vi "Main.vi"(11 "Module Admin":refnum<class "Delacor_lib_QMH_Module Admin.lvclass">) -> ()   [LabVIEW 2021, in "Test Panel.lvlib"]
doc: "This template is based off of the Queued Message Handler design pattern and the Queued Message Handler project template that ships with LabVIEW.\n\nThe main difference is that the queue is private to this module and communication between modules is performed via Broadcast and Request events.\n\nRequest events are wrapped in public API methods and are handled in the Event Handling Loop (EHL) of this VI. Any module can register for Broadcast events sent by this module. The EHL generates messages based on user interface actions.\n\nThe Message Handling Loop (MHL) processes messages generated by the EHL, or by other messages. The messages are string values, so new messages can be added easily to the Message Cases case structure in the MHL. Each message cluster can also provide an optional value for Message Data, which is a variant that can be converted to whatever message-specific data is required.\n_____\nBased on DQMH Project Template 7.0.1.1316."
uses:
  Test Panel.lvlib
  <vilib>/Delacor/Delacor QMH/Libraries/Module Admin_class/Delacor_lib_QMH_Module Admin.lvclass
  Module Data--cluster.ctl
  GUI Ctrl Data's--Cluster.ctl
  Rx-Mapping Data.ctl
  <vilib>/Wovalab/Utilities/Helper Loop Periodic Timing/Helper Loop Periodic Timing.lvclass/Helper Loop Periodic Timing.ctl
  Host-Control's/Module ID Action Enum.ctl
  <vilib>/Delacor/Delacor QMH/Libraries/Message Queue_class/Delacor_lib_QMH_Message Queue.lvclass/Delacor_lib_QMH_Message Queue.ctl
  Digital Output/Controls/DO Update Cluster.ctl
  Stop Argument--cluster.ctl
  <vilib>/Delacor/Delacor QMH/Libraries/Module Admin_class/Delacor_lib_QMH_Module Admin.lvclass/Delacor_lib_QMH_Module Admin.ctl
  <vilib>/Utility/miscctls.llb/LVPointTypeDef.ctl
  Host-Control's/HW Name Enum.ctl
  <vilib>/Delacor/Delacor QMH/Libraries/Message Queue_class/Delacor_lib_QMH_Enqueue Message (Single).vi
  <vilib>/Delacor/Delacor QMH/Libraries/Module Admin_class/Delacor_lib_QMH_Get External Launch.vi
  <vilib>/Wovalab/Utilities/Helper Loop Periodic Timing/U32 Max Value--constant.vi
  <vilib>/Wovalab/Utilities/Helper Loop Periodic Timing/Update Last Execution Time.vi
  <vilib>/addons/_JKI.lib/Serialization/JSON/Library/Flatten To JSON String.vi
  <vilib>/Wovalab/Utilities/Helper Loop Periodic Timing/Helper Loop Periodic Timing.lvclass
  <vilib>/Delacor/Delacor QMH/Libraries/Message Queue_class/Delacor_lib_QMH_Message Queue.lvclass
  RT Acquisition Engine/RT Acquisition Engine.lvlib
  Main-Module/Host Main.lvlib
  <userlib>/_OpenG.lib/appcontrol/appcontrol.llb/openg_application_control.lvlib
  Hardware Selection/Hardware Selection.lvlib
  Test Panel GUI Update/Test Panel GUI Update.lvlib
panel:
  out "MFC Value's":T1
  out "Thermocouple Value's":T2
  out "AI-Channel Data's":dbl[](array[numeric])
  out "AI-Time":string
  out "AI-Channels":string[](array[string])
  out "Capsule-4":bool
  out "Capsule-3":bool
  out "Capsule-2":bool
  out "Time":string
  out "Data":bool[](array[boolean])
  out "Channels":string[](array[string])
  out "Drop Time":string
  in  "Gate valve Delay (mS)":u32=1000
  in  "EM valve Delay (mS)":u32=1000
  out "Auto Status":string
  out "12":dbl
  out "15":dbl
  out "16":dbl
  out "11":dbl
  out "14":dbl
  out "13":dbl
  out "8":dbl caption="Nichrome + S*2"
  out "7":dbl caption="Nichrome + S*1"
  out "6":dbl caption="Light S*2"
  out "10":dbl caption="Cam Trigger S*2"
  out "9":dbl caption="Cam Trigger S*1"
  out "5":dbl caption="Light S*1"
  out "4":dbl caption="Nichrome - S*2"
  out "3":dbl caption="Nichrome - S*1"
  out "2":dbl caption="Fan S*2"
  out "1":dbl caption="Fan S*1"
  in  "Sec Fan":bool
  out "Nicrome + 2":bool caption="Nichrome +"
  out "Current":dbl
  out "Diff":dbl
  out "Auto Seq":u8
  in  "Camera Trig. Delay(ms)":u32=50
  in  "Camera Trigger Delay(s)":bool=TRUE
  in  "Camera Power Off Delay(s)":u32
  out "Cam Trig from Release":bool
  out "Release Er No.":i32
  out "Safety Er No.":i32
  out "Proximity Status":string
  in  "Proximity_Disable":bool
  out "Status 2":string
  in  "Fan":bool
  in  "Cam Power":bool
  in  "Ground Clearance":dbl format="%#_13g"
  in  "Count down":dbl=7.0
  out "Pressure Signal 1":dbl format="%#_4g"
  out "Airbag Pressure":dbl format="%0#_4g"
  out "Gate Valve- Right 2":bool
  out "Gate Valve- Left":bool
  in  "Electro Magnet Lid-Right":bool
  in  "Electro Magnet Lid-Left":bool
  in  "Gate Valve-Left":bool
  in  "Gate Valve- Right":bool
  in  "Distance":dbl
  out "Ground Reference":dbl(slide) scale=0.0..500.0
  in  "Secondary Camera":bool
  in  "Motion Studio":bool
  in  "Stop":bool caption="Start_"
  out "NiCr Continuity":bool
  out "Safety":enum16{"Dis-Engaged by User", "Engaged"}(ring)
  out "Experimental":enum16{"Dis-Engaged by User", "Engaged"}(ring)
  out "Release":enum16{"Dis-Engaged by User", "Engaged"}(ring)
  out "SAFETY":bool
  out "RELEASE":bool
  out "SB-RIO":bool
  out "Capsule-1":bool
  out "Test Progress":bool
  out "Elapsed Time":dbl
  out "Message":string
  in  "Safety Valve_Switch":bool caption="Sensor power"
  in  "Check for Proceed":bool
  in  "Primary Camera":bool
  in  "Nicrome Status":bool
  in  "Saftey and Release":bool
  in  "Numeric":dbl
  out "Captured":bool
  out "Capture Time":timestamp
  out "Proximity 2":timestamp
  out "Start Time":timestamp
  out "Proximity":bool
  in  "Cam Trigger":bool
  in  "Nicrome -":bool caption="Nichrome -"
  in  "Nicrome +":bool caption="Nichrome +"
  in  "Light":bool
  in  "Sensor power":bool caption="Sensor Power"
  in  "Enable":bool
  out "Safety Sensor 3":bool
  out "Safety Sensor 2":bool
  out "Safety Sensor 1":bool
  out "Unlock Sensor":bool
  out "Lock Sensor":bool
  in  "Release Valve Control":bool caption="Sensor power"
  out "Valve 1":bool
  out "Valve 2":bool
  out "Valve 3":bool
  out "Release Valve":bool
  in  "Start":bool caption="Sensor power"
  out "Drag Shield Refernce":dbl(slide) scale=0.0..500.0
  out "error out 2":errorcluster
  out "error out":errorcluster
  out "Status":string
  in  "Simulate MHL Error":bool
  in  "Simulate EHL Error":bool
  # "IIT M Drop Tower Test System"
  # "MIMIC PANEL"
  # "STATUS"
  # "USER CHECK LIST"
  # "DROP CONTROL"
  # "Safety And Release"
  # "Circuit Status"
  # "Primary camera"
  # "Secondary camera"
  # "Check To Proceed"
  # "RELEASE"
  # "SAFETY"
  # "Experimental Capsule Parameters"
  # "DROP CAPSULE STATUS"
  # "AIRBAG CONTROLLER"
  # "Gate valve and Electromagnet Control"
  # "Gate valve Status"
  # "Pressure Indicator"
  # "In mm"
  # "m"
  # "In mm"
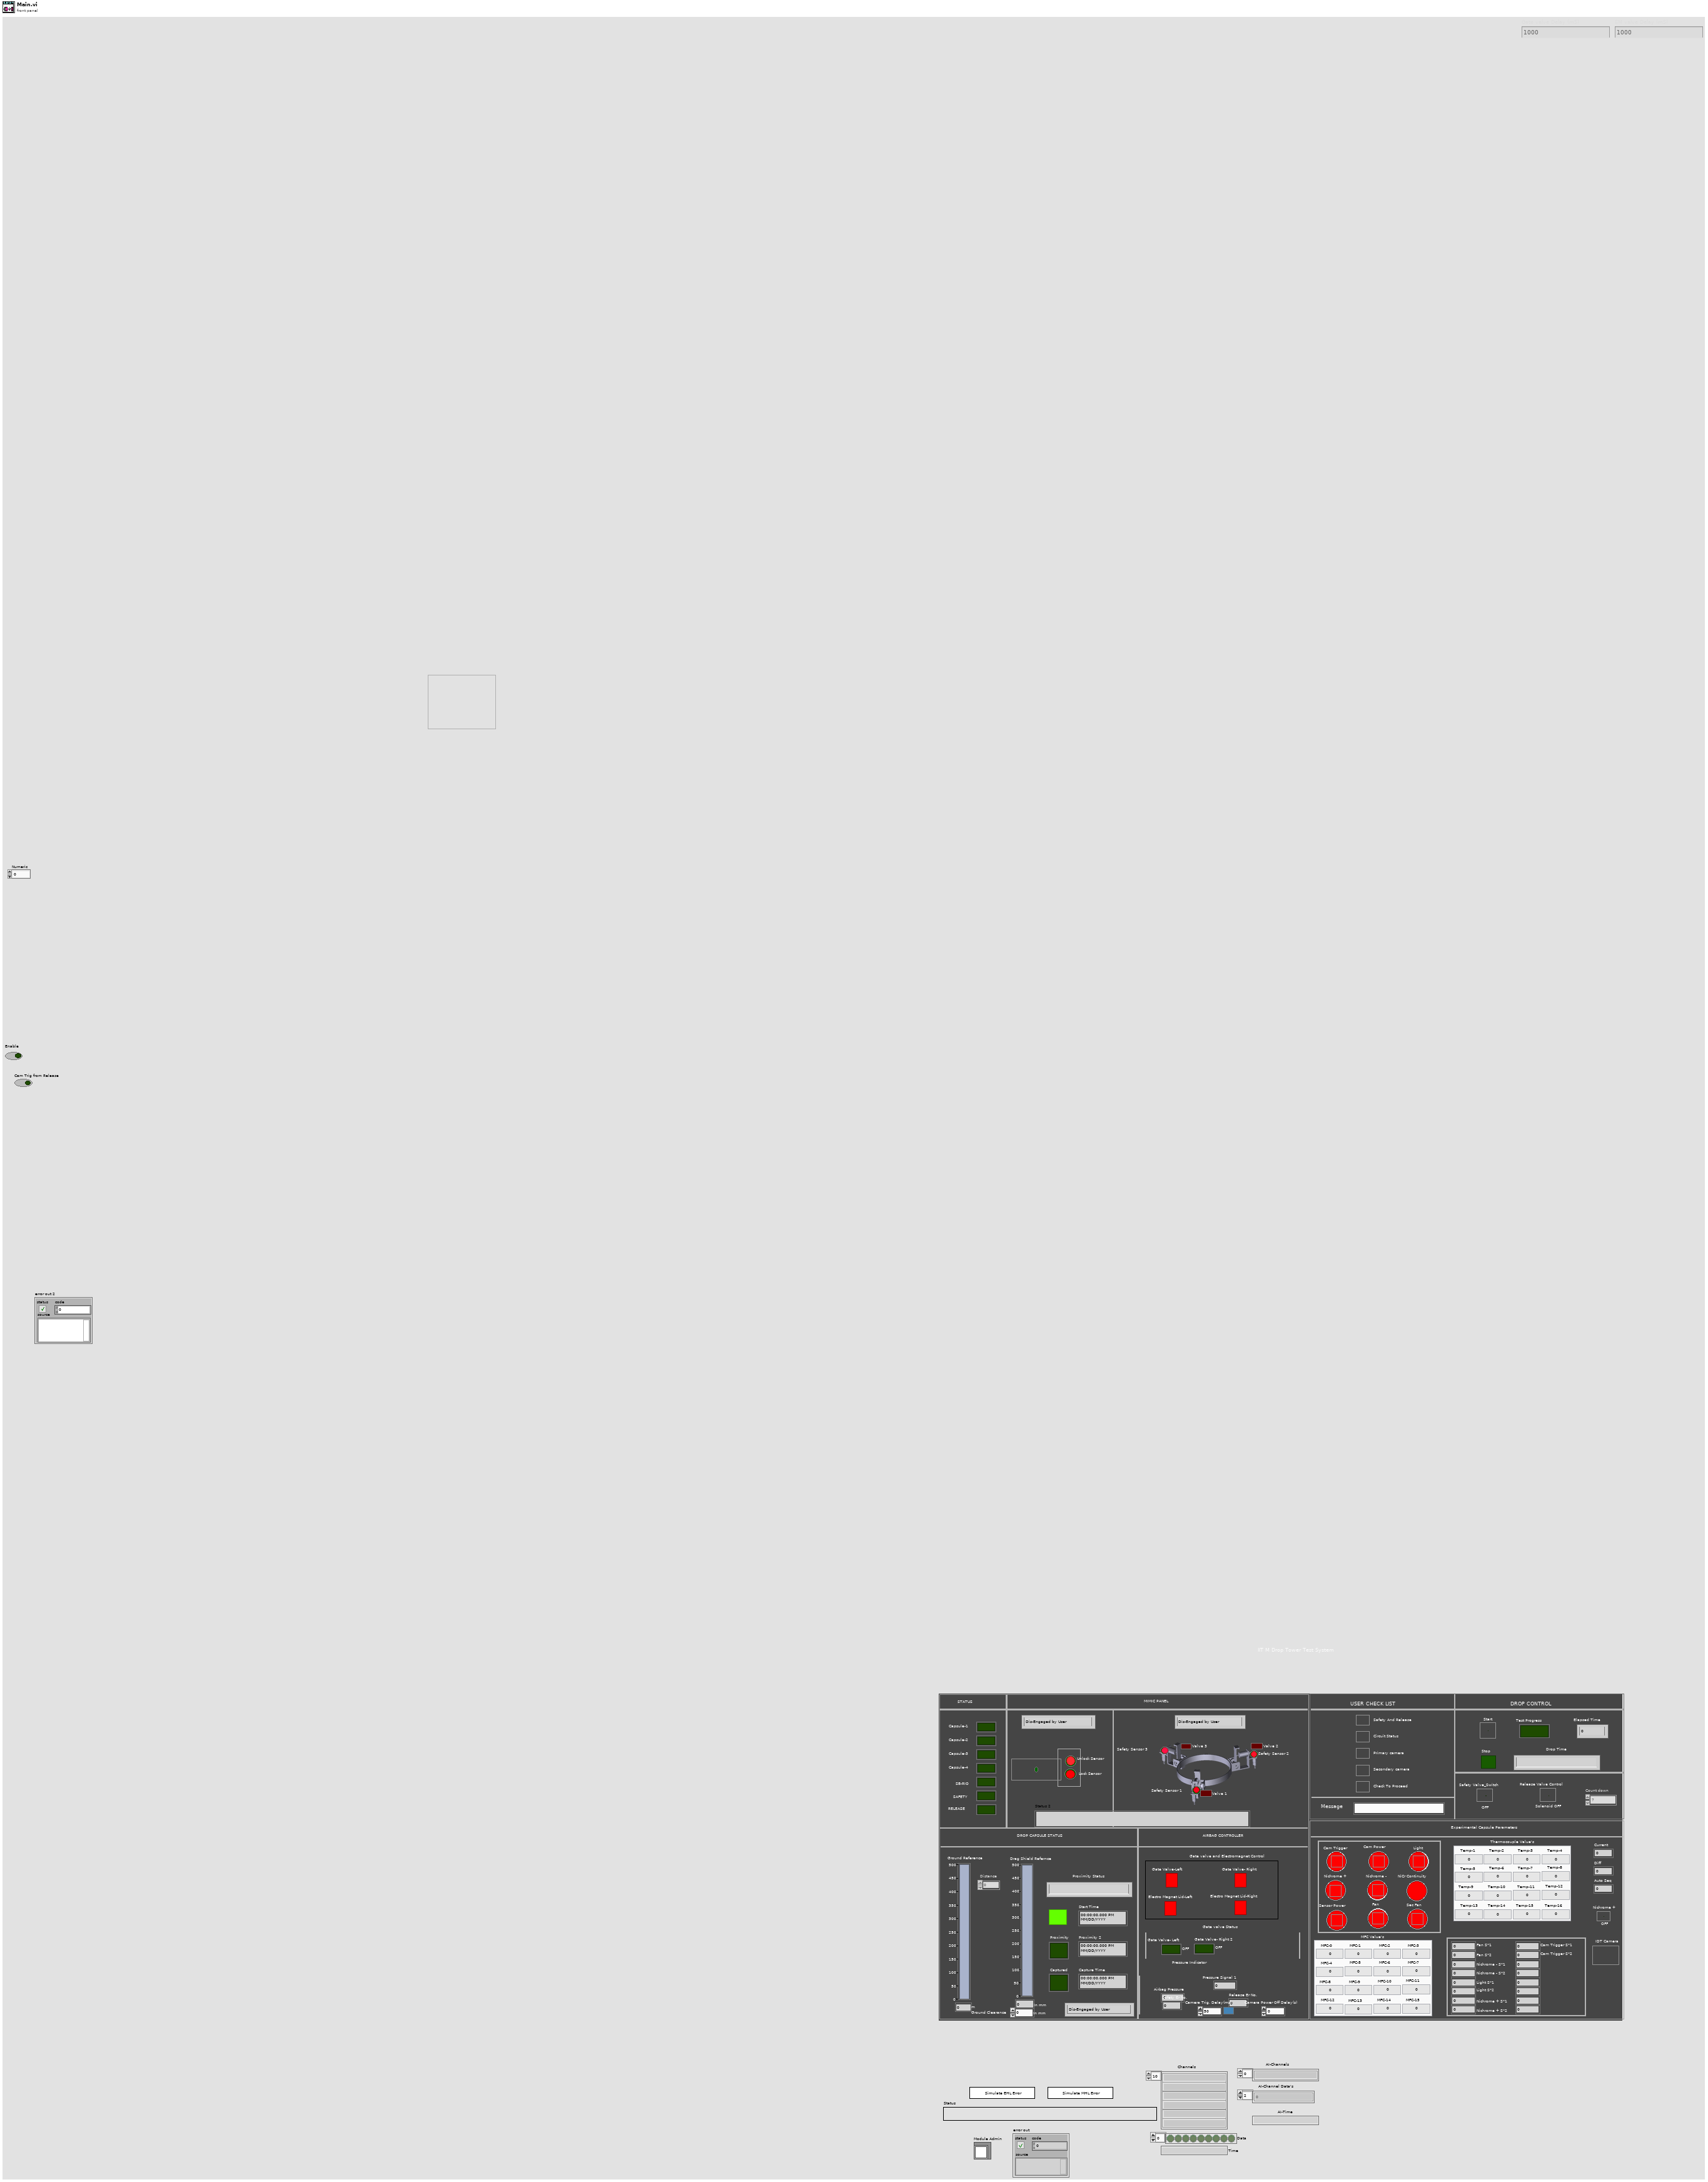
[diagram p1: front panel]
types:
  T1 = cluster{"MFC-0":dbl, "MFC-1":dbl, "MFC-2":dbl, "MFC-3":dbl, "MFC-4":dbl, "MFC-5":dbl, "MFC-6":dbl, "MFC-7":dbl, "MFC-8":dbl, "MFC-9":dbl, "MFC-10":dbl, "MFC-11":dbl, "MFC-12":dbl, "MFC-13":dbl, "MFC-14":dbl, "MFC-15":dbl}
  T2 = cluster{"Temp-1":dbl, "Temp-2":dbl, "Temp-3":dbl, "Temp-4":dbl, "Temp-5":dbl, "Temp-6":dbl, "Temp-7":dbl, "Temp-8":dbl, "Temp-9":dbl, "Temp-10":dbl, "Temp-11":dbl, "Temp-12":dbl, "Temp-13":dbl, "Temp-14":dbl, "Temp-15":dbl, "Temp-16":dbl}
  T3 = typedef "Test Panel.lvlib/Request Events--cluster.ctl" = cluster{"Stop Module":refnum<user-event>, "Show Panel":refnum<user-event>, "Hide Panel":refnum<user-event>, "Get Module Execution Status":refnum<user-event>, "Show Diagram":refnum<user-event>}
  T4 = typedef "Test Panel.lvlib/Module Data--cluster.ctl" = cluster{"Status":string, "RT-HW-Data":cluster{"RT-HW-Name":string[], "RT-HW-IP":string[]}, "Pane":refnum<vi>, "Tx-Maping Data":string[][], "GUI Ctrl Data's":T5, "Rx-Mapping Data":T6, "This VI":refnum<vi>}
  T5 = typedef "Test Panel.lvlib/GUI Ctrl Data's--Cluster.ctl" = cluster{"All Ctrl and Indi Label":string[], "All Ctrl & Indi Ref":refnum<vi>[]}
  T6 = typedef "Test Panel.lvlib/Rx-Mapping Data.ctl" = cluster{"Mapped Ctrl and Indi Label":string[], "Mapped Hardware Name":string[], "Mapped Interface Name":string[], "Mapped Channel Name":string[]}
  T7 = typedef "Module ID Action Enum.ctl" = enum16{"Init", "Insert", "Get a ID", "Get all ID"}
  T8 = cluster{"RT-HW-Name":string[], "RT-HW-IP":string[]}
  T9 = typedef "DO Update Cluster.ctl" = cluster{"Channel":string[], "Data":u8[]}
  T10 = enum32{"invalid lock state", "Not Locked", "Locked (No Password)", "Password-protected"}
  T11 = typedef "Test Panel.lvlib/Stop Argument--cluster.ctl" = cluster{"Origin":string, "Exit via Stop Module Req?":bool, "Wait for Module to stop?":bool}
  T12 = typedef "LVPointTypeDef.ctl" = cluster{"Horizontal":i16, "Vertical":i16}
  T13 = enum32{"Invalid", "Standard", "Closed", "Hidden", "Minimized", "Maximized"}
  T14 = typedef "HW Name Enum.ctl" = enum16{"Capsule-1", "Capsule-2", "Capsule-3", "Capsule-4", "sb-RIO", "Safety", "Release"}
  T15 = typedef "Test Panel GUI Update.lvlib/Broadcast Events--cluster.ctl" = cluster{"Module Did Init":refnum<user-event>, "Status Updated":refnum<user-event>, "Error Reported":refnum<user-event>, "Module Did Stop":refnum<user-event>, "Update Module Execution Status":refnum<user-event>}
  T16 = typedef "RT Acquisition Engine.lvlib/Broadcast Events--cluster.ctl" = cluster{"Module Did Init":refnum<user-event>, "Status Updated":refnum<user-event>, "Error Reported":refnum<user-event>, "Module Did Stop":refnum<user-event>, "Update Module Execution Status":refnum<user-event>, "RT Connection Status":refnum<user-event>, "Tx RT Hardware Info":refnum<user-event>, "DO Data's":refnum<user-event>, "AI-Info":refnum<user-event>}
  T17 = typedef "Host Main.lvlib/Broadcast Events--cluster.ctl" = cluster{"Module Did Init":refnum<user-event>, "Status Updated":refnum<user-event>, "Error Reported":refnum<user-event>, "Module Did Stop":refnum<user-event>, "Update Module Execution Status":refnum<user-event>, "RT-Module Id's":refnum<user-event>}
  T18 = typedef "Hardware Selection.lvlib/Broadcast Events--cluster.ctl" = cluster{"Module Did Init":refnum<user-event>, "Status Updated":refnum<user-event>, "Error Reported":refnum<user-event>, "Module Did Stop":refnum<user-event>, "Update Module Execution Status":refnum<user-event>, "Selected RT HW":refnum<user-event>}
  T19 = typedef "DIO Data's from RT.ctl" = cluster{"Channels":string[], "Data":bool[], "Time":string}
  T20 = typedef "AI-Data from RT.ctl" = cluster{"Channel Name's":string[], "Channel Data's":dbl[], "Date & Time":string}
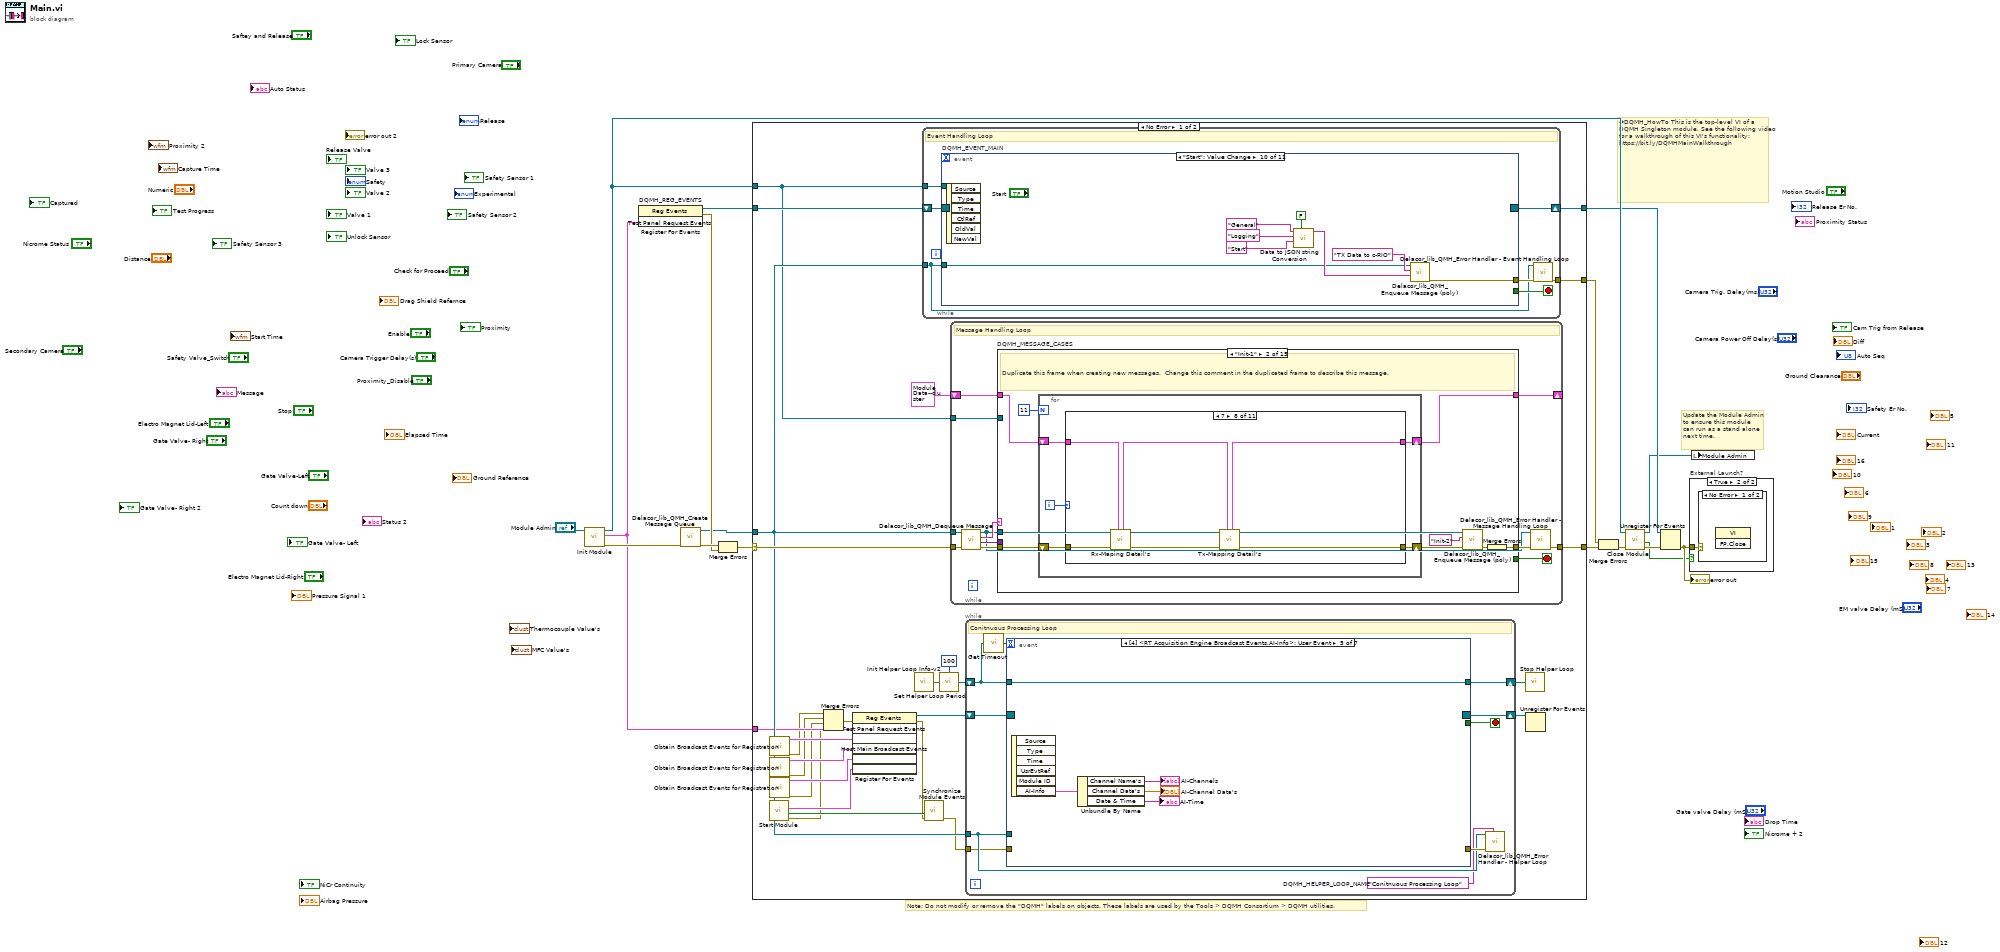
[diagram p0: block diagram]
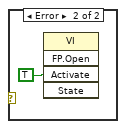
[diagram p3: hidden frame]
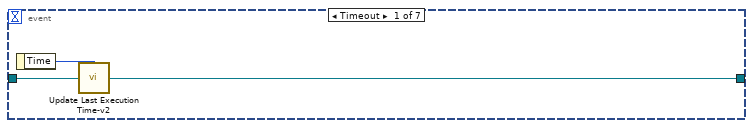
[diagram p4: hidden frame]
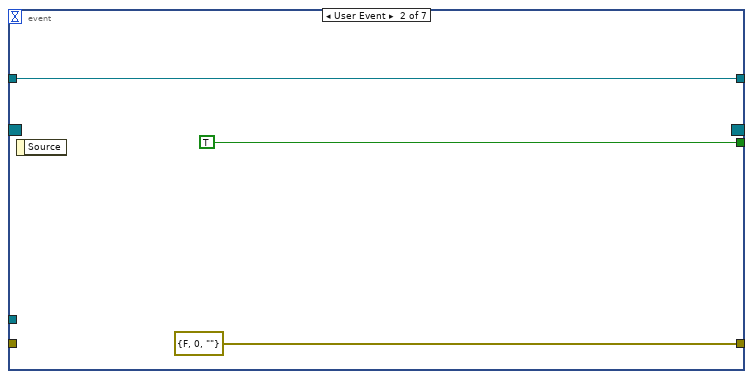
[diagram p5: hidden frame]
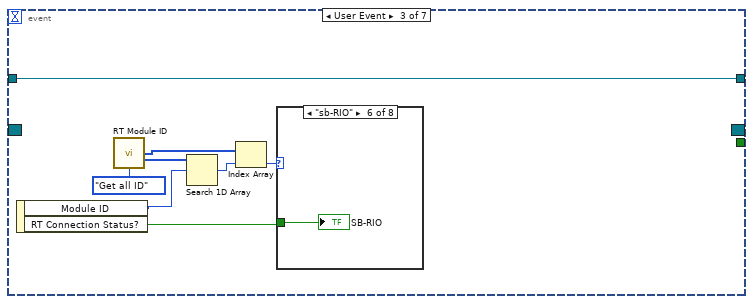
[diagram p6: hidden frame]
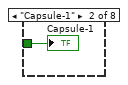
[diagram p8: hidden frame]
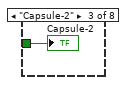
[diagram p9: hidden frame]
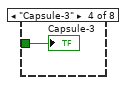
[diagram p10: hidden frame]
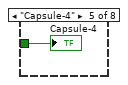
[diagram p11: hidden frame]
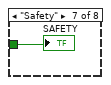
[diagram p12: hidden frame]
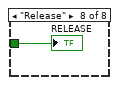
[diagram p13: hidden frame]
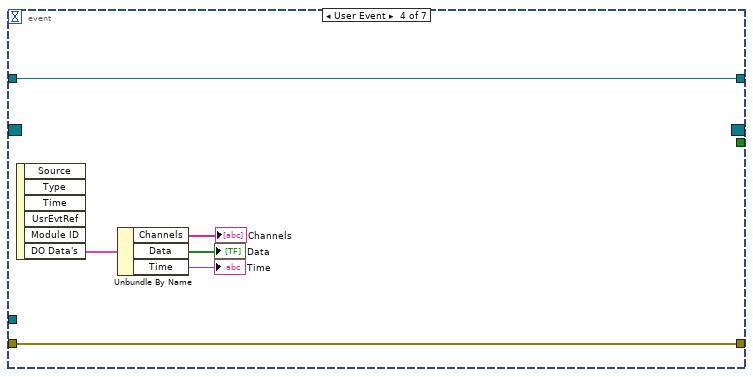
[diagram p14: hidden frame]
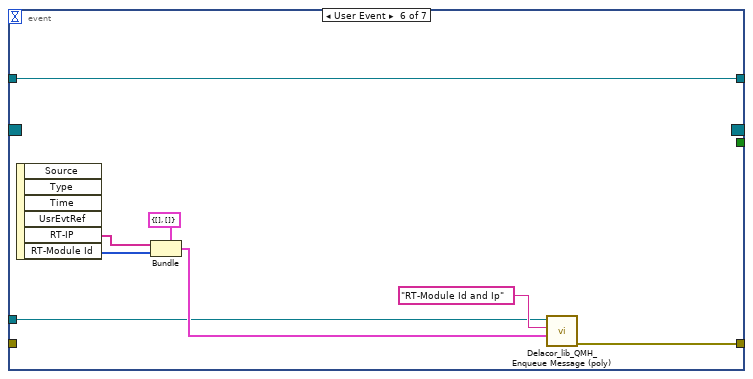
[diagram p15: hidden frame]
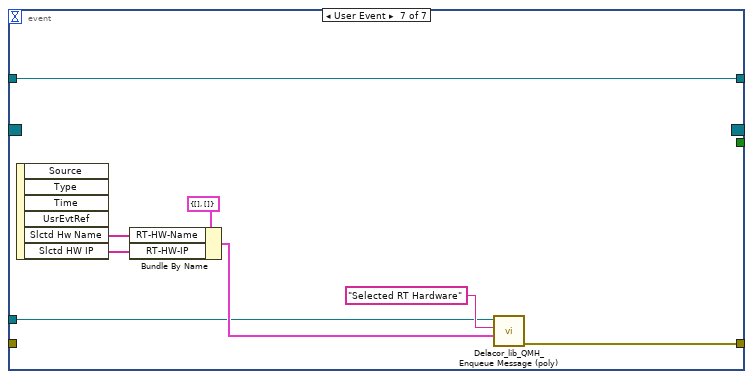
[diagram p16: hidden frame]
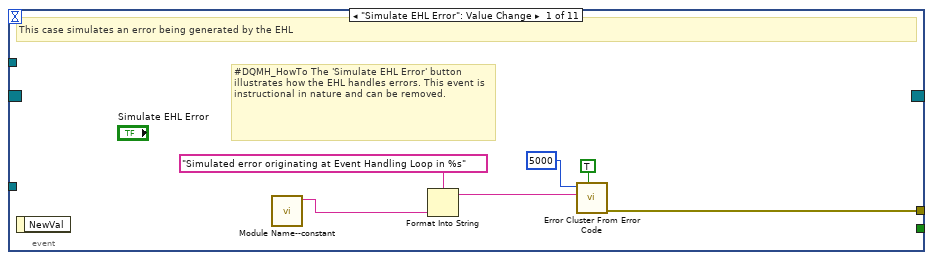
[diagram p17: hidden frame]
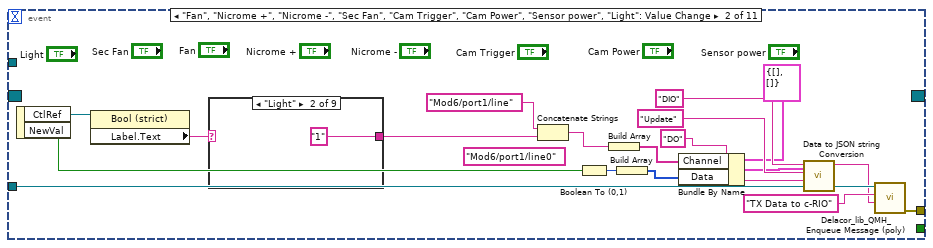
[diagram p18: hidden frame]
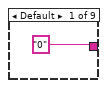
[diagram p19: hidden frame]
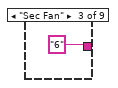
[diagram p20: hidden frame]
diagram:
  # "#DQMH_HowTo This is the top-level VI of a DQMH Singleton module. See the following video for a walkthrough of this VI's functionality: https://bit.ly/DQMHMainWalkthrough"
  # "Note: Do not modify or remove the \"DQMH\" labels on objects. These labels are used by the Tools > DQMH Consortium > DQMH utilities."
  # "Update the Module Admin to ensure this module can run as a stand alone next time."
  n1 = call "Init Module.vi"("Singleton Module Admin in"="Module Admin") -> ("error out"=w16:errorcluster, "Test Panel Request Events"=w1:T3, "Singleton Module Admin out"=w8:refnum<class "Delacor_lib_QMH_Module Admin.lvclass">)  [unwired: 8 in]
  n2 = register-events "DQMH_REG_EVENTS"(w1) -> (reference out=w6:refnum<event-registration>, error out=w9:errorcluster)  [unwired: 2 in]
  n3 = call <vilib>:"Delacor_lib_QMH_Create Message Queue.vi"("error in"=w16) -> ("error out"=w11:errorcluster, "Message Queue"=w5:refnum<class "Delacor_lib_QMH_Message Queue.lvclass">)  [unwired: 9 in]
  n4 = Merge Errors(w11, w9) -> (w10:errorcluster)
  n5 = case shown="No Error" w10 {
    selector: w10 -> [w42 w409]
    tunnel: [w44 w408] -> w17
    tunnel: [w41 w407] -> w7
    tunnel: w6 -> [w39 w407]
    tunnel: w5 -> [w38 w402]
    tunnel: [w43 _] -> w14
    tunnel: w8 -> [w37 w403]
    tunnel: w1 -> [w36 _]
    frame No Error {
      n6 = call "Start Module.vi"() -> ("error out"=w18:errorcluster, "Wait for Event Sync?"=w25:bool, "Test Panel GUI Update Broadcast Events"=w26:T15)  [unwired: 8 in, 1 out]
      n7 = call "Obtain Broadcast Events for Registration.vi"() -> ("error out"=w21:errorcluster, "RT Acquisition Engine Broadcast Events"=w29:T16)  [unwired: 9 in, 1 out]
      n8 = call "Obtain Broadcast Events for Registration.vi"() -> ("error out"=w20:errorcluster, "Host Main Broadcast Events"=w28:T17)  [unwired: 9 in, 1 out]
      n9 = call "Obtain Broadcast Events for Registration.vi"() -> ("error out"=w19:errorcluster, "Hardware Selection Broadcast Events"=w27:T18)  [unwired: 9 in, 1 out]
      n10 = Merge Errors(w21, w20, w19, w18) -> (w22:errorcluster)
      n11 = register-events ("DQMH_HELPER_REGFOREVENTS")(error in=w22, w36, w29, w28, w27, w26) -> (reference out=w34:refnum<event-registration>, error out=w24:errorcluster)  [unwired: 1 in]
      n12 = call <vilib>:"Init Helper Loop Info-v2.vi"() -> ("Helper Loop Periodic Timing"=w31:refnum<class "Helper Loop Periodic Timing.lvclass">)  [unwired: 1 in]
      n13 = while {
        tunnel: w38 -> [w103]
        shift-right: [w106] -> w41
        shift-left: w39 -> [w107]
        tunnel: [w108] -> w43
        tunnel: w37 -> [w104]
        stop <- w105 stop-if-true
        # "Event Handling Loop"
        n14 = event "DQMH_EVENT_MAIN" shown="[9] \"Start\": Value Change" {
          selector: w107 -> [_ _ _ _ _ _ _ _ _ _ _]
          dyn-events: [_ _ _ _ _ _ _ _ _ _ _] -> w106
          timeout: _ -> [_ _ _ _ _ _ _ _ _ _ _]
          tunnel: [_ _ _ _ _ _ _ TRUE ("Discard?") _ _ _] -> w105
          tunnel: w103 -> [_ w129 w144 _ _ _ _ w163 w180 w183 w193]
          tunnel: [w115 w130 w145 _ _ w151 _ w173 w181 w184 w195] -> w109
          tunnel: w104 -> [_ _ _ _ _ _ _ _ _ _ w192]
          event "Simulate EHL Error": Value Change {
            # "#DQMH_HowTo The 'Simulate EHL Error' button  illustrates how the EHL handles errors. This event is instructional in nature and can be removed."
            # "This case simulates an error being generated by the EHL"
            n15 = event-data() -> ()  [unwired: 1 in, 1 out]
            n16 = call "Module Name--constant.vi"() -> ("Module Name"=w112:string)  [unwired: 11 in]
            n17 = Format Into String(format string="Simulated error originating at Event Handling Loop in %s", w112) -> (resulting string=w113:string)  [unwired: 2 in, 1 out]
            n18 = call <vilib>:"Error Cluster From Error Code.vi"("show call chain? (False)"=TRUE, "error message (\"\")"=w113, "error code (0)"=5000) -> ("error out"=w115:errorcluster)  [unwired: 6 in]
          }
          event "Fan", "Nicrome +", "Nicrome -", "Sec Fan", "Cam Trigger", "Cam Power", "Sensor power", "Light": Value Change {
            (unwired) "Mod6/port1/line0" ("String")
            n19 = event-data() -> ("CtlRef"=w128:refnum<vi>, "NewVal"=w133:bool)  [unwired: 1 in]
            n20 = property class="Bool (strict)"(reference=w128) -> ("Label.Text"=w127:string)  [unwired: 1 in, 2 out]
            n21 = case shown="\"Light\"" w127 {
              tunnel: ["0" "1" "6" "5" "2" "3" "5" "4" "0"] -> w125
              frame Default {
              }
              frame "Light" {
              }
              frame "Sec Fan" {
              }
              frame "Fan" {
              }
              frame "Nicrome +" {
              }
              frame "Nicrome -" {
              }
              frame "Cam Trigger" {
              }
              frame "Cam Power" {
              }
              frame "Sensor power" {
              }
            }
            n22 = Concatenate Strings("Mod6/port1/line" ("String"), w125) -> (w124:string)
            n23 = Boolean To (0,1)(Boolean=w133) -> (0, 1=w132:i16)
            n24 = Build Array(w124) -> (w118:string[])
            n25 = Build Array(w132) -> (w117:i16[])
            n26 = Bundle By Name(cluster=T9 {"Channel"=[], "Data"=[]} ("DO Update Cluster"), "Channel"=w118, "Data"=w117) -> (w116:T9)
            n27 = call "Data to JSON string Conversion.vi"("Data"=w116, "SubCmd"="DO" ("Interface Data.SubCmd"), "Command"="Update" ("Interface Data.Command"), "Interface"="DIO") -> ("Cmd String"=w120:string)  [unwired: 6 in, 1 out]
            n28 = call-poly <vilib>:"Delacor_lib_QMH_Enqueue Message (poly).vi"("Message Data"=w120, "Message"="TX Data to c-RIO", "Message Queue in"=w129) -> ("error out"=w130:errorcluster)  [unwired: 7 in, 1 out]
          }
          event "Simulate MHL Error": Value Change {
            # "#DQMH_HowTo The 'Simulate MHL Error' button  illustrates how the MHL handles errors. This event is instructional in nature and can be removed."
            # "This case simulates an error being generated by the MHL"
            n29 = event-data() -> ()  [unwired: 1 in, 1 out]
            n30 = call-poly <vilib>:"Delacor_lib_QMH_Enqueue Message (poly).vi"("Message"="Simulate MHL Error", "Message Queue in"=w144) -> ("error out"=w145:errorcluster)  [unwired: 8 in, 1 out]
          }
          event User Event {
            # "Show the panel of this VI, and send a status updated message to let listeners know."
            # "Another Module called the \"Show Panel\" API Method."
            n31 = event-data() -> ()  [unwired: 1 in, 1 out]
            n32 = control-ref of="This VI"() -> (w147:refnum<vi>)
            n33 = call "Open VI Panel.vi"("VI"=w147) -> ()  [unwired: 10 in, 1 out]
            n34 = call "Status Updated.vi"("Status"="Panel shown." ("format string")) -> ()  [unwired: 10 in, 1 out]
          }
          event User Event {
            # "Hide the panel of this VI, and send a status updated message to let listeners know."
            # "Another Module called the \"Hide Panel\" API Method."
            n35 = event-data() -> ()  [unwired: 1 in, 1 out]
            n36 = control-ref of="This VI"() -> (w149:refnum<vi>)
            n37 = call "Hide VI Panel.vi"("VI"=w149) -> ()  [unwired: 10 in, 1 out]
            n38 = call "Status Updated.vi"("Status"="Panel hidden." ("format string")) -> ()  [unwired: 10 in, 1 out]
          }
          event User Event {
            # "Another Module called the \"Get Module Execution Status\" API Method."
            n39 = event-data() -> ()  [unwired: 1 in, 1 out]
            n40 = call "Update Module Execution Status.vi"("Running?"=TRUE) -> ("error out"=w151:errorcluster)  [unwired: 10 in]
          }
          event User Event {
            # "Another Module called the \"Show Diagram\" API Method. This event is used for debugging."
            n41 = event-data() -> ()  [unwired: 1 in, 1 out]
            n42 = disable-structure shown="RUN_TIME_ENGINE==False" {
              frame condition #0 (active) {
                # "functionality not available in exe"
                n43 = invoke on="Invoke Node" class="VI" method="Lock State.Get"() -> (error out=w157:errorcluster, "Get Lock State"=w156:T10, "pwd in cache"=w153:bool)  [unwired: 4 in, 1 out]
                n44 = Equal?(x=T10."Password-protected", y=w156) -> (x = y?=w154:bool)
                n45 = Compound Arithmetic op=AND(w154, invert w153) -> (w152:bool)
                n46 = case shown="False" w152 {
                  tunnel: w157 -> [w160 _]
                  frame False {
                    n47 = property on="Property Node" class="VI"(error in=w160, "BDWin.Open"=TRUE ("Block Diagram Window:Open")) -> ()  [unwired: 1 in, 2 out]
                    n48 = call "Status Updated.vi"("Status"="Block Diagram shown." ("format string")) -> ()  [unwired: 10 in, 1 out]
                  }
                  frame True {
                    # "Password-protected VI, and the password is not in the cache. Do not show the diagram."
                  }
                }
              }
              frame condition #1 {
              }
            }
          }
          event User Event {
            # "The Stop Module Event can get fired from the Exit message in the MHL. The queue gets destroyed in that case. If the queue no longer exists, the Enqueue Exit as a priority message will return error 1. It is safe to ignore, because the module is already exiting."
            # "Another Module called the \"Stop Module\" API Method  or the Message Handling Loop below."
            n49 = event-data() -> ("Origin"=w170:string, "Exit via Stop Module Req?"=w166:bool, "Wait for Module to stop?"=w165:bool)  [unwired: 1 in]
            n50 = local write "Status"(w170) -> ()
            n51 = Bundle By Name(cluster=T11 {"Origin"="", "Exit via Stop Module Req?"=FALSE, "Wait for Module to stop?"=FALSE} ("Stop Argument"), "Exit via Stop Module Req?"=w166, "Wait for Module to stop?"=w165) -> (w164:T11)
            n52 = call-dynamic "Delacor_lib_QMH_Flush Messages.vi"("Message Queue in"=w163) -> ("error out"=w161:errorcluster, "Message Queue out"=w162:refnum<class "Delacor_lib_QMH_Message Queue.lvclass">)  [unwired: 7 in, 2 out]
            n53 = call-poly <vilib>:"Delacor_lib_QMH_Enqueue Message (poly).vi"("Priority Message? (F)"=TRUE, "error in"=w161, "Message Data"=w164, "Message"="Exit", "Message Queue in"=w162) -> ("error out"=w174:errorcluster)  [unwired: 5 in, 1 out]
            n54 = call <vilib>:"Clear Errors.vi"("error in (no error)"=w174, "specific error code to clear (0: all)"=1) -> ("error out"=w173:errorcluster)  [unwired: 4 in, 1 out]
          }
          event "Release Valve Control": Value Change {
            n55 = event-data() -> ()  [unwired: 1 in, 3 out]
            n56 = call "Data to JSON string Conversion.vi"("Data"=FALSE, "SubCmd"="Start", "Command"="AutoSequence", "Interface"="General") -> ("Cmd String"=w179:string)  [unwired: 6 in, 1 out]
            n57 = call-poly <vilib>:"Delacor_lib_QMH_Enqueue Message (poly).vi"("Message Data"=w179, "Message"="TX Data to c-RIO", "Message Queue in"=w180) -> ("error out"=w181:errorcluster)  [unwired: 7 in, 1 out]
          }
          event "Start": Value Change {
            n58 = event-data() -> ()  [unwired: 1 in, 6 out]
            n59 = call "Data to JSON string Conversion.vi"("Data"=FALSE, "SubCmd"="Start", "Command"="Logging", "Interface"="General") -> ("Cmd String"=w189:string)  [unwired: 6 in, 1 out]
            n60 = call-poly <vilib>:"Delacor_lib_QMH_Enqueue Message (poly).vi"("Message Data"=w189, "Message"="TX Data to c-RIO", "Message Queue in"=w183) -> ("error out"=w184:errorcluster)  [unwired: 7 in, 1 out]
          }
          event Panel Close? {
            w194 = TRUE  # Discard the event, the MHL is responsible for closing and stopping this VI.
            # "Hide the panel or send the 'Exit' message if the user clicks the 'X' on the module main VI panel."
            n61 = event-data() -> ()  [unwired: 1 in, 1 out]
            n62 = property on="Property Node" class="Module Admin"(reference=w192) -> ("Accessors:External Launch"=w191:bool)  [unwired: 1 in, 2 out]
            n63 = case shown="False" w191 {
              tunnel: w193 -> [w201 w208]
              tunnel: [w197 w211] -> w195
              frame True {
                # "If externally launched, clicking the 'X' hides the panel, but doesn't close it."
                n64 = control-ref of="This VI"() -> (w205:refnum<vi>)
                n65 = call "Hide VI Panel.vi"("VI"=w205) -> ("error out"=w203:errorcluster)  [unwired: 10 in]
                n66 = call "Status Updated.vi"("error in"=w203, "Status"="Panel hidden." ("format string")) -> ("error out"=w200:errorcluster)  [unwired: 9 in]
                n67 = call-dynamic "Delacor_lib_QMH_Flush Messages.vi"("error in"=w200, "Message Queue in"=w201) -> ("error out"=w198:errorcluster, "Message Queue out"=w199:refnum<class "Delacor_lib_QMH_Message Queue.lvclass">)  [unwired: 6 in, 2 out]
                n68 = call-poly <vilib>:"Delacor_lib_QMH_Enqueue Message (poly).vi"("Priority Message? (F)"=TRUE, "error in"=w198, "Message"="Exit", "Message Queue in"=w199) -> ("error out"=w197:errorcluster)  [unwired: 6 in, 1 out]
              }
              frame False {
                # "If run as a stand-alone VI, clicking the panel 'X' stops the VI."
                n69 = call-dynamic "Delacor_lib_QMH_Flush Messages.vi"("Message Queue in"=w208) -> ("error out"=w206:errorcluster, "Message Queue out"=w207:refnum<class "Delacor_lib_QMH_Message Queue.lvclass">)  [unwired: 7 in, 2 out]
                n70 = call-poly <vilib>:"Delacor_lib_QMH_Enqueue Message (poly).vi"("Priority Message? (F)"=TRUE, "error in"=w206, "Message"="Exit", "Message Queue in"=w207) -> ("error out"=w211:errorcluster)  [unwired: 6 in, 1 out]
              }
            }
            n71 = event-data ("Event Filter Node")("Discard?"=w194) -> ()  [unwired: 1 in, 1 out]
          }
        }
        n72 = call-dynamic "Delacor_lib_QMH_Error Handler - Event Handling Loop.vi"("error in"=w109, "Message Queue in"=w103) -> ("dup error in"=w108:errorcluster)  [unwired: 8 in, 1 out]
      }
      n73 = call "Synchronize Module Events.vi"("error in"=w24, "Wait for Event Sync?"=w25) -> ("error out"=w23:errorcluster)  [unwired: 9 in]
      n74 = call <vilib>:"Set Helper Loop Period.vi"("Period (ms)"=100, "Helper Loop Periodic Timing in"=w31) -> ("Helper Loop Periodic Timing out"=w33:refnum<class "Helper Loop Periodic Timing.lvclass">)  [unwired: 13 in]
      n75 = while {
        tunnel: w38 -> [w212]
        shift-right: [w220] -> _
        shift-left: T4 {"Status"="", "RT-HW-Data"={"RT-HW-Name"=[], "RT-HW-IP"=[]}, "Pane"=refnum, "Tx-Maping Data"=[], "GUI Ctrl Data's"={"All Ctrl and Indi Label"=[], "All Ctrl & Indi Ref"=[]}, "Rx-Mapping Data"={"Mapped Ctrl and Indi Label"=[], "Mapped Hardware Name"=[], "Mapped Interface Name"=[], "Mapped Channel Name"=[]}, "This VI"=refnum} ("Data Cluster") -> [w221]
        tunnel: w42 -> [w223]
        tunnel: [w215] -> w44
        tunnel: w37 -> [w216]
        stop <- w219 stop-if-true
        # "Message Handling Loop"
        n76 = call-dynamic "Delacor_lib_QMH_Dequeue Message.vi"("error in"=w223, "Message Queue in"=w212) -> ("error out"=w222:errorcluster, "Message Data"=w217:variant, "Message"=w218:string, "Message Queue out"=w213:refnum<class "Delacor_lib_QMH_Message Queue.lvclass">)  [unwired: 6 in]
        n77 = case "DQMH_MESSAGE_CASES" shown="\"Init-1\"" w218 {
          selector: w218 -> [_ _ _ _ _ _ _ _ _ _ _ _ _ _ w397]
          tunnel: w213 -> [w225 w255 _ _ _ _ _ _ _ w338 _ _ w362 w385 _]
          tunnel: w222 -> [w246 w251 w300 w302 w304 w307 w309 w315 w324 w347 w349 w358 w369 w391 w400]
          tunnel: [w226 w257 w299 w302 w304 w306 w312 w314 w326 w339 w349 w357 w365 w386 w401] -> w214
          tunnel: w221 -> [w236 w250 w298 w301 w303 w305 w311 w313 w323 w345 w348 w355 w364 w384 w398]
          tunnel: [w235 w249 w298 w301 w303 w305 w310 w313 w323 w344 w348 w355 w364 w384 w398] -> w220
          tunnel: [_ _ _ _ _ _ _ _ _ _ _ _ _ w383 _] -> w219
          tunnel: w217 -> [_ _ _ _ _ _ _ _ w325 w346 _ _ w363 w382 _]
          tunnel: w216 -> [w237 _ _ _ _ _ _ _ _ _ _ _ w361 w377 _]
          frame "Initialize" {
            w231 = "Initial Message" ("Initial Message")
            # "#CodeNeeded - Initialize the appearance of the front panel."
            # "#CodeNeeded - Initialize your state data here."
            # "Initialize - Any operation that needs to be done before the module can receive messages. Synchronize Caller Events.vi will inform Start Module.vi that the module has launched and is ready to receive messages. Module Did Init.vi will broadcast that the module initialized."
            n78 = call "Synchronize Caller Events.vi"("error in"=w246, "Singleton Module Admin in"=w237) -> ("error out"=w245:errorcluster, "Singleton Module Admin out"=w232:refnum<class "Delacor_lib_QMH_Module Admin.lvclass">)  [unwired: 8 in]
            n79 = property on="Property Node" class="Module Admin"(reference=w232) -> ("Accessors:External Launch"=w241:bool)  [unwired: 1 in, 2 out]
            n80 = Select(t=T13."Hidden" ("State"), s=w241, f=T13."Standard" ("State")) -> (s? t:f=w238:T13)
            n81 = control-ref of="This VI"() -> (w224:refnum<vi>)
            n82 = call "Module Name--constant.vi"() -> ("Module Name"=w244:string)  [unwired: 11 in]
            n83 = property on="Property Node" class="VI"(reference=w224, "Front Panel.Title"=w244) -> (reference out=w243:refnum<vi>, error out=w248:errorcluster)  [unwired: 1 in]
            n84 = call "Module Name--constant.vi"() -> ("Module Name"=w233:string)  [unwired: 11 in]
            n85 = invoke on="Invoke Node" class="VI" method="FP.Open"(reference=w243, error in=w248, "State"=w238) -> (reference out=w242:refnum<vi>, error out=w247:errorcluster)  [unwired: 2 in, 3 out]
            n86 = Bundle By Name(cluster=w236, "Status"=w231) -> (w235:T4)
            n87 = call "Module Did Init.vi"("error in"=w245, "Initialized?"=TRUE, "Origin"=w233) -> ("error out"=w227:errorcluster)  [unwired: 8 in]
            n88 = invoke on="Invoke Node" class="VI" method="FP.Center"(reference=w242, error in=w247) -> ()  [unwired: 1 in, 3 out]
            n89 = property on="Pane" class="Pane"("Origin"=T12 {"Horizontal"=0, "Vertical"=0}) -> ()  [unwired: 2 in, 2 out]
            n90 = call <userlib>:"Fit VI window to Largest Dec__ogtk.vi"() -> ("error out"=w229:errorcluster)  [unwired: 6 in, 1 out]
            n91 = call <vilib>:"Clear Errors.vi"("error in (no error)"=w229) -> ()  [unwired: 5 in, 2 out]
            n92 = call-poly <vilib>:"Delacor_lib_QMH_Enqueue Message (poly).vi"("error in"=w227, "Message"="Init-1", "Message Queue in"=w225) -> ("error out"=w226:errorcluster)  [unwired: 7 in, 1 out]
            "Status" <- w231
          }
          frame "Init-1" {
            # "Duplicate this frame when creating new messages.  Change this comment in the duplicated frame to describe this message."
            n93 = for {
              N: 11 -> [_]
              shift-right: [w261] -> w252
              shift-left: w251 -> [w260]
              shift-right: [w258] -> w249
              shift-left: w250 -> [w259]
              i -> [w262]
              n94 = case shown="7" w262 {
                tunnel: [w267 w269 w270 w276 w279 w281 w283 w284 w292 w295 w297] -> w261
                tunnel: w260 -> [w267 w269 w271 w277 w279 w281 w283 w288 w293 w295 w297]
                tunnel: w259 -> [w266 w268 w273 w275 w278 w280 w282 w289 w291 w294 w296]
                tunnel: [w265 w268 w272 w275 w278 w280 w282 w286 w291 w294 w296] -> w258
                frame 0, Default {
                  # "Reference's are taken and bundled in this data cluster."
                  n95 = control-ref of="This VI"() -> (w263:refnum<vi>)
                  n96 = control-ref of="Pane"() -> (w264:refnum<vi>)
                  n97 = Bundle By Name(cluster=w266, "Pane"=w264, "This VI"=w263) -> (w265:T4)
                }
                frame 1 {
                  # "Reference's are taken and bundled in this data cluster."
                }
                frame 2 {
                  n98 = call "Seperating Reference and Label.vi"("Data Cluster In"=w273, "error in (no error)"=w271) -> ("error out"=w270:errorcluster, "Data Cluster Out"=w272:T4)  [unwired: 8 in]
                }
                frame 3 {
                  # "Send the Ctrl ref and Ctrl Label to the GUI Update Module"
                  n99 = Unbundle By Name(w275) -> ("GUI Ctrl Data's"=w274:T5)
                  n100 = call "Get GUI Ctrl Data.vi"("error in"=w277, "GUI Ctrl Data's"=w274) -> ("error out"=w276:errorcluster)  [unwired: 9 in]
                }
                frame 4 {
                }
                frame 5 {
                }
                frame 6 {
                }
                frame 7 {
                  n101 = call "Rx-Maping Detail's.vi"("Data Cluster In"=w289, "error in (no error)"=w288) -> ("error out"=w285:errorcluster, "Data Cluster Out"=w287:T4)  [unwired: 8 in]
                  n102 = call "Tx-Mapping Detail's.vi"("Data Cluster In"=w287, "error in (no error)"=w285) -> ("error out"=w284:errorcluster, "Data Cluster Out"=w286:T4)  [unwired: 8 in]
                }
                frame 8 {
                  # "Transmit Rx-Mapping Data to the GUI Update Module"
                  n103 = Unbundle By Name(w291) -> ("Rx-Mapping Data"=w290:T6)
                  n104 = call "Get GUI Mapping Data's.vi"("error in"=w293, "Mapping Deatils"=w290) -> ("error out"=w292:errorcluster)  [unwired: 9 in]
                }
                frame 9 {
                }
                frame 10 {
                }
              }
            }
            n105 = call-poly <vilib>:"Delacor_lib_QMH_Enqueue Message (poly).vi"("error in"=w252, "Message"="Init-2", "Message Queue in"=w255) -> ("error out"=w256:errorcluster)  [unwired: 7 in, 1 out]
            n106 = Merge Errors(w256) -> (w257:errorcluster)
          }
          frame "Init-2" {
            # "Duplicate this frame when creating new messages.  Change this comment in the duplicated frame to describe this message."
            n107 = call "Get Selected RT Hardware.vi"() -> ()  [unwired: 11 in, 1 out]
            n108 = Merge Errors(w300) -> (w299:errorcluster)
          }
          frame "---Module Specific---" {
            # "Separator -- The following cases handle messages specific to this Module."
          }
          frame "Send Data to Hardware" {
            # "Separator -- The following cases handle messages specific to this Module."
          }
          frame "---Copy This Frame---" {
            # "Duplicate this frame when creating new messages.  Change this comment in the duplicated frame to describe this message."
            n109 = Merge Errors(w307) -> (w306:errorcluster)
          }
          frame "Start All RT Engine" {
            # "Duplicate this frame when creating new messages.  Change this comment in the duplicated frame to describe this message."
            n110 = call "Send Start Command to RT Hardware's.vi"("Data Cluster In"=w311, "error in (no error)"=w309) -> ("error out"=w308:errorcluster, "Data Cluster Out"=w310:T4)  [unwired: 8 in]
            n111 = Merge Errors(w308) -> (w312:errorcluster)
          }
          frame "Configure All RT Engine" {
            # "Duplicate this frame when creating new messages.  Change this comment in the duplicated frame to describe this message."
            n112 = disable-structure shown="Disabled" {
              frame Disabled {
                w317 = u16 0 items=["192.168.32.50", "192.168.32.15"] ("RT-IP")
                n113 = call "Host - Configuration to command.vi"() -> ()  [unwired: 10 in, 2 out]
                n114 = call "RT Module ID.vi"("Action"=w317) -> ("Module Id Out"=w316:i32)  [unwired: 11 in, 3 out]
                n115 = call "Write Data To the RT.vi"("Module ID"=w316) -> ()  [unwired: 10 in, 1 out]
              }
              frame Enabled {
              }
            }
            n116 = Merge Errors(w315) -> (w314:errorcluster)
          }
          frame "TX Data to c-RIO" {
            # "Duplicate this frame when creating new messages.  Change this comment in the duplicated frame to describe this message."
            n117 = Unbundle By Name(w323) -> ("RT-HW-Data.RT-HW-Name"=w321:string[])
            n118 = Variant To Data(error in=w324, type="", Variant=w325) -> (data=w319:string, error out=w320:errorcluster)
            n119 = for {
              tunnel: w321 -> [w330] mode=indexing
              tunnel: w319 -> [w327]
              shift-right: [w328] -> w318
              shift-left: w320 -> [w329]
              n120 = case shown="\"Capsule-4\"" w330 {
                tunnel: w329 -> [w331 w337]
                tunnel: [w331 w336] -> w328
                tunnel: w327 -> [_ w335]
                frame "False", Default {
                }
                frame "Capsule-4" {
                  n121 = call "RT Module ID.vi"("HW Name"=HW_Name_Enum."Capsule-4", "Action"=Module_ID_Action_Enum."Get a ID") -> ("Module Id Out"=w334:i32)  [unwired: 10 in, 3 out]
                  n122 = call "Write Data To the RT.vi"("error in"=w337, "Data In"=w335, "Module ID"=w334) -> ("error out"=w336:errorcluster)  [unwired: 8 in]
                }
              }
            }
            n123 = Merge Errors(w318) -> (w326:errorcluster)
          }
          frame "Selected RT Hardware" {
            n124 = Variant To Data(error in=w347, type=T8 {"RT-HW-Name"=[], "RT-HW-IP"=[]}, Variant=w346) -> (data=w342:T8, error out=w340:errorcluster)
            n125 = Bundle By Name(cluster=w345, "RT-HW-Data"=w342) -> (w344:T4)
            n126 = call-poly <vilib>:"Delacor_lib_QMH_Enqueue Message (poly).vi"("error in"=w340, "Message"="Start All RT Engine", "Message Queue in"=w338) -> ("error out"=w339:errorcluster)  [unwired: 7 in, 1 out]
          }
          frame "---Exit and Error Handling---" {
            # "Separator - The following cases handle errors and exit messages."
          }
          frame "Simulate MHL Error" {
            # "#DQMH_HowTo The 'Simulate MHL Error' button  illustrates how the MHL handles errors. This event is instructional in nature and can be removed."
            # "Simulate an error occurring at the MHL"
            n127 = call "Module Name--constant.vi"() -> ("Module Name"=w351:string)  [unwired: 11 in]
            n128 = Format Into String(format string="Simulated error originating at Message Handling Loop in %s", w351) -> (resulting string=w352:string)  [unwired: 2 in, 1 out]
            n129 = call <vilib>:"Error Cluster From Error Code.vi"("show call chain? (False)"=TRUE, "error message (\"\")"=w352, "error code (0)"=5001) -> ("error out"=w356:errorcluster)  [unwired: 6 in]
            n130 = Merge Errors(w358, w356) -> (w357:errorcluster)
          }
          frame "Error" {
            # "#CodeRecommended - If the module is running in standalone mode (External Launch = FALSE), this code will pop up an error dialog and call the 'Exit' message if an error occurs. Add more fine-grained error management here."
            # "Error - Check the error message data and respond accordingly. This message is sent by the \"Error Handler\" VIs at the end of each loop in this application."
            n131 = Variant To Data(error in=w369, type=errorcluster {"status"=FALSE, "code"=0, "source"=""} ("error constant"), Variant=w363) -> (data=w359:errorcluster, error out=w367:errorcluster)
            n132 = property on="Property Node" class="Module Admin"(reference=w361) -> ("Accessors:External Launch"=w360:bool)  [unwired: 1 in, 2 out]
            n133 = local write "error out"(w359) -> ()
            n134 = call "Error Reported.vi"("Error"=w359) -> ()  [unwired: 10 in, 1 out]
            n135 = case shown="False" w360 {
              tunnel: [w374 _] -> w366
              tunnel: w362 -> [w372 _]
              tunnel: w359 -> [w373 _]
              frame False {
                n136 = disable-structure shown="Default" {
                  disable-tunnel: w373 -> [w375 _]
                  frame condition #0 (active) {
                    # "If the module is running standalone, then pop up an error dialog and call the \"Exit\" message."
                    n137 = call <vilib>:"Simple Error Handler.vi"("error in (no error)"=w375) -> ()  [unwired: 4 in, 5 out]
                  }
                  frame condition #1 {
                    # "To prevent the Simple Error Handler VI from being loaded (e.g. when deploying to a Real-Time target), add the Conditional Disable Symbol \"DQMH_Disable_SEH\" to your project and set it to TRUE."
                  }
                }
                n138 = call-poly <vilib>:"Delacor_lib_QMH_Enqueue Message (poly).vi"("Priority Message? (F)"=TRUE, "Message"="Exit", "Message Queue in"=w372) -> ("error out"=w374:errorcluster)  [unwired: 7 in, 1 out]
              }
              frame True {
                # "If the module was launched externally, calling the Error Reported broadcast VI is the only action performed by the \"Error\" message. The module's caller can then process the error appropriately."
              }
            }
            n139 = Merge Errors(w367, w366) -> (w365:errorcluster)
          }
          frame "Exit" {
            w381 = 91  # 91: not all Exit messages will have an argument
            w383 = TRUE  # Stop the VI
            # "Release the message queue reference"
            # "#CodeNeeded - Add any required cleanup code here."
            # "Exit - Exit the application."
            n140 = Variant To Data(error in=w391, type=T11 {"Origin"="", "Exit via Stop Module Req?"=FALSE, "Wait for Module to stop?"=FALSE} ("Stop Argument"), Variant=w382) -> (data=w379:T11, error out=w388:errorcluster)
            n141 = call <vilib>:"Clear Errors.vi"("error in (no error)"=w388, "specific error code to clear (0: all)"=w381) -> ("error out"=w390:errorcluster)  [unwired: 4 in, 1 out]
            n142 = control-ref of="This VI"() -> (w378:refnum<vi>)
            n143 = call "Handle Exit.vi"("Stop Argument"=w379, "Admin in"=w377, "VI reference"=w378) -> ("error out"=w387:errorcluster)  [unwired: 7 in, 1 out]
            n144 = call-dynamic "Delacor_lib_QMH_Release Message Queue.vi"("error in"=w390, "Message Queue"=w385) -> ("error out"=w389:errorcluster)  [unwired: 9 in]
            n145 = Merge Errors(w389, w387) -> (w386:errorcluster)
            n146 = call "Error Reported.vi"("Error"=w386) -> ()  [unwired: 10 in, 1 out]
            n147 = call "Stop Module.vi"() -> ("error out"=w376:errorcluster)  [unwired: 11 in]
            n148 = call "Show Panel.vi"("error in"=w376) -> ()  [unwired: 10 in, 1 out]
          }
          frame Default {
            # "'Default' case only runs if there is a message that isn't defined in any of the other cases.  Output a programming error."
            n149 = call "Module Name--constant.vi"() -> ("Module Name"=w396:string)  [unwired: 11 in]
            n150 = Format Into String(format string="The invalid message string \"%s\" was received in the Message Handling Loop for module \"%s\".", w397, w396) -> (resulting string=w392:string)  [unwired: 2 in, 1 out]
            n151 = call <vilib>:"Error Cluster From Error Code.vi"("show call chain? (False)"=TRUE, "error message (\"\")"=w392, "error code (0)"=1) -> ("error out"=w399:errorcluster)  [unwired: 6 in]
            n152 = Merge Errors(w400, w399) -> (w401:errorcluster)
          }
        }
        n153 = call-dynamic "Delacor_lib_QMH_Error Handler - Message Handling Loop.vi"("error in"=w214, "Message Queue in"=w213) -> ("dup error in"=w215:errorcluster)  [unwired: 8 in, 1 out]
      }
      n154 = while "DQMH_HELPER_LOOP" {
        shift-right: [w54] -> w32
        shift-left: w33 -> [w46]
        shift-right: [w52] -> w35
        shift-left: w34 -> [w53]
        tunnel: w38 -> [w49]
        tunnel: w23 -> [w45]
        stop <- w51 stop-if-true
        w48 = "Conitnuous Processing Loop"  # DQMH_HELPER_LOOP_NAME
        # "Conitnuous Processing Loop"
        n155 = call <vilib>:"Get Timeout.vi"("Helper Loop Periodic Timing"=w46) -> ("Timeout (ms)"=w47:i32)  [unwired: 12 in, 2 out]
        n156 = event "DQMH_HELPER_EVENT_STRUCTURE" shown="[4] <RT Acquisition Engine Broadcast Events.AI-Info>: User Event" {
          selector: w53 -> [_ _ _ _ _ _ _]
          dyn-events: [_ _ _ _ _ _ _] -> w52
          timeout: w47 -> [_ _ _ _ _ _ _]
          tunnel: w46 -> [w56 w60 w68 w81 w86 w94 w102]
          tunnel: [w55 w60 w68 w81 w86 w94 w102] -> w54
          tunnel: [_ TRUE _ _ _ _ _] -> w51
          tunnel: [_ errorcluster {"status"=FALSE, "code"=0, "source"=""} ("error constant") _ w76 _ w87 w95] -> w50
          tunnel: w49 -> [_ _ _ _ _ w88 w96]
          tunnel: w45 -> [_ _ _ w76 _ _ _]
          event Timeout {
            n157 = event-data() -> ("Time"=w57:u32)  [unwired: 1 in]
            n158 = call <vilib>:"Update Last Execution Time-v2.vi"("Time"=w57, "Helper Loop Periodic Timing in"=w56) -> ("Helper Loop Periodic Timing out"=w55:refnum<class "Helper Loop Periodic Timing.lvclass">)  [unwired: 12 in, 1 out]
          }
          event User Event {
            n159 = event-data() -> ()  [unwired: 1 in, 1 out]
          }
          event User Event {
            n160 = event-data() -> ("Module ID"=w62:i32, "RT Connection Status?"=w61:bool)  [unwired: 1 in]
            n161 = call "RT Module ID.vi"("Action"=Module_ID_Action_Enum."Get all ID") -> ("All HW Name Out"=w64:T14[], "All HW-ID Out"=w65:i32[])  [unwired: 11 in, 2 out]
            n162 = Search 1D Array(1D array=w65, element=w62) -> (index of element=w66:i32)  [unwired: 1 in]
            n163 = Index Array(array=w64, index=w66) -> (element=w63:T14)
            n164 = case shown="\"sb-RIO\"" w63 {
              tunnel: w61 -> [_ w69 w70 w71 w72 w73 w74 w75]
              frame Default {
              }
              frame "Capsule-1" {
                "Capsule-1" <- w69
              }
              frame "Capsule-2" {
                "Capsule-2" <- w70
              }
              frame "Capsule-3" {
                "Capsule-3" <- w71
              }
              frame "Capsule-4" {
                "Capsule-4" <- w72
              }
              frame "sb-RIO" {
                "SB-RIO" <- w73
              }
              frame "Safety" {
                "SAFETY" <- w74
              }
              frame "Release" {
                "RELEASE" <- w75
              }
            }
          }
          event User Event {
            n165 = event-data() -> ("DO Data's"=w80:T19)  [unwired: 1 in, 5 out]
            n166 = Unbundle By Name(w80) -> ("Channels"=→"Channels":string[], "Data"=→"Data":bool[], "Time"=→"Time":string)
          }
          event User Event {
            n167 = event-data() -> ("AI-Info"=w83:T20)  [unwired: 1 in, 5 out]
            n168 = Unbundle By Name(w83) -> ("Channel Name's"=→"AI-Channels":string[], "Channel Data's"=→"AI-Channel Data's":dbl[], "Date & Time"=→"AI-Time":string)
          }
          event User Event {
            n169 = event-data() -> ("RT-IP"=w91:string[], "RT-Module Id"=w90:i32[])  [unwired: 1 in, 4 out]
            n170 = Bundle(cluster=cluster{"RT-IP":string[], "RT-Module Id":i32[]} {"RT-IP"=[], "RT-Module Id"=[]}, "RT-IP"=w91, "RT-Module Id"=w90) -> (w89:cluster{"RT-IP":string[], "RT-Module Id":i32[]})
            n171 = call-poly <vilib>:"Delacor_lib_QMH_Enqueue Message (poly).vi"("Message Data"=w89, "Message"="RT-Module Id and Ip", "Message Queue in"=w88) -> ("error out"=w87:errorcluster)  [unwired: 7 in, 1 out]
          }
          event User Event {
            n172 = event-data() -> ("Slctd Hw Name"=w100:string[], "Slctd HW IP"=w99:string[])  [unwired: 1 in, 4 out]
            n173 = Bundle By Name(cluster=T8 {"RT-HW-Name"=[], "RT-HW-IP"=[]}, "RT-HW-Name"=w100, "RT-HW-IP"=w99) -> (w97:T8)
            n174 = call-poly <vilib>:"Delacor_lib_QMH_Enqueue Message (poly).vi"("Message Data"=w97, "Message"="Selected RT Hardware", "Message Queue in"=w96) -> ("error out"=w95:errorcluster)  [unwired: 7 in, 1 out]
          }
        }
        n175 = call-dynamic "Delacor_lib_QMH_Error Handler - Helper Loop.vi"("Error Debug"=w48, "error in"=w50, "Message Queue in"=w49) -> ()  [unwired: 7 in, 2 out]
      }
      n176 = call <vilib>:"Stop Helper Loop.vi"("Helper Loop Periodic Timing in"=w32) -> ()  [unwired: 1 out]
      n177 = Unregister For Events(event registration refnum=w35) -> ()  [unwired: 1 in, 1 out]
    }
    frame Error {
      # "Synchronize Caller Events.vi will inform Start Module.vi that the module has launched and will let the code calling Start Module.vi register for broadcasts and would permit the caller receive the broadcast that an error occurred at launch time."
      n178 = call-dynamic "Delacor_lib_QMH_Release Message Queue.vi"("error in"=w409, "Message Queue"=w402) -> ("error out"=w408:errorcluster)  [unwired: 9 in]
      n179 = call "Synchronize Caller Events.vi"("Singleton Module Admin in"=w403) -> ("error out"=w410:errorcluster)  [unwired: 9 in, 1 out]
      n180 = call "Module Name--constant.vi"() -> ("Module Name"=w406:string)  [unwired: 11 in]
      n181 = Format Into String(format string="An error occurred during initialization. %s is no longer running.", w406) -> (resulting string=w404:string)  [unwired: 2 in, 1 out]
      n182 = Merge Errors(w408, w410) -> (w411:errorcluster)
      n183 = call "Error Reported.vi"("Additional Information"=w404, "Error"=w411) -> ()  [unwired: 9 in, 1 out]
    }
  }
  n184 = Merge Errors(w14, w17) -> (w13:errorcluster)
  n185 = call "Close Module.vi"("error in"=w13, "Module Admin in"=w8) -> ("error out"=w15:errorcluster, "External Launch"=w2:bool, "Module Admin out"=w3:refnum<class "Delacor_lib_QMH_Module Admin.lvclass">)  [unwired: 7 in]
  n186 = Unregister For Events(event registration refnum=w7, error in=w15) -> (error out=w12:errorcluster)
  "error out" <- w12
  n187 = case "External Launch?" shown="True" w2 {
    tunnel: w12 -> [_ w412]
    frame False {
    }
    frame True {
      n188 = case shown="No Error" w412 {
        frame No Error {
          n189 = invoke on="Invoke Node" class="VI" method="FP.Close"() -> ()  [unwired: 3 in, 3 out]
        }
        frame Error {
          n190 = invoke on="Invoke Node" class="VI" method="FP.Open"("Activate"=TRUE ("Activate?")) -> ()  [unwired: 4 in, 5 out]
        }
      }
    }
  }
  n191 = local write "Module Admin"(w3) -> ()
